vi "2 Global.vi"() -> ()   [LabVIEW 2011]
uses:
  2 Typedefs/UTM Location.ctl
  2 Typedefs/apparent wind.ctl
  2 Typedefs/apparent wind speed.ctl
  2 Typedefs/apparent wind direction.ctl
  2 Typedefs/Velocity.ctl
  2 Typedefs/heading.ctl
  2 Typedefs/generalized actuator status.ctl
  2 Typedefs/indicator LED.ctl
  2 Typedefs/generalized sensor status.ctl
  2 Typedefs/Which Boat.ctl
  2 Typedefs/manual override.ctl
  2 Typedefs/setpoints to boat.ctl
  2 Typedefs/sail setpt.ctl
  2 Typedefs/rudder angle.ctl
panel:
  in  "E-Stop":bool
  in  "Globals":T1(tab)
  in  "Which Boat Am I?":T2 items=["Small RC", "Large RC", "Final Boat", "Simulator"]
  out "Direction Sensor Status":T3
  out "Location Sensor Status":T3
  out "Wind Sensor Status":T3
  out "Sail Actuator Status":T5
  out "Rudder Actuator Status":T5
  in  "Battery Voltage":dbl
  in  "Robot\nHeading":T6 format="%05.1f"
  in  "Robot UTM Location":T7
  in  "Robot Velocity":T8
  out "Overview Image":T9(plugin-control)
  in  "Absolute Wind":T8
  in  "Apparent Wind\nDirection":T10
  in  "Apparent Wind\nSpeed":T11
  in  "Apparent Wind":T12
  in  "Current Destination":T7
  in  "Setpoints to boat":T13
  in  "Manual Override Cluster":T16
  in  "Sail Position":T14
  in  "Rudder Angle":T15
  # "All distances in meters, all speeds in meters per second\nAll angles in degrees, clockwise with 0 being positive North if in global reference frame or 0 being Fore in boat ref frame.\nX-Y make a right handed coordinate system with Z pointing up\nPositive Rudder angle makes the boat turn right\nLocation Coordinates are in UTM format"
  # "As Measured"
  # "From Planning Functions"
  # "Path Planning"
  # "(this is not a cluster because subitems\nare generated in parallel code)"
  # "Mission Definition Stuff Goes HERE"
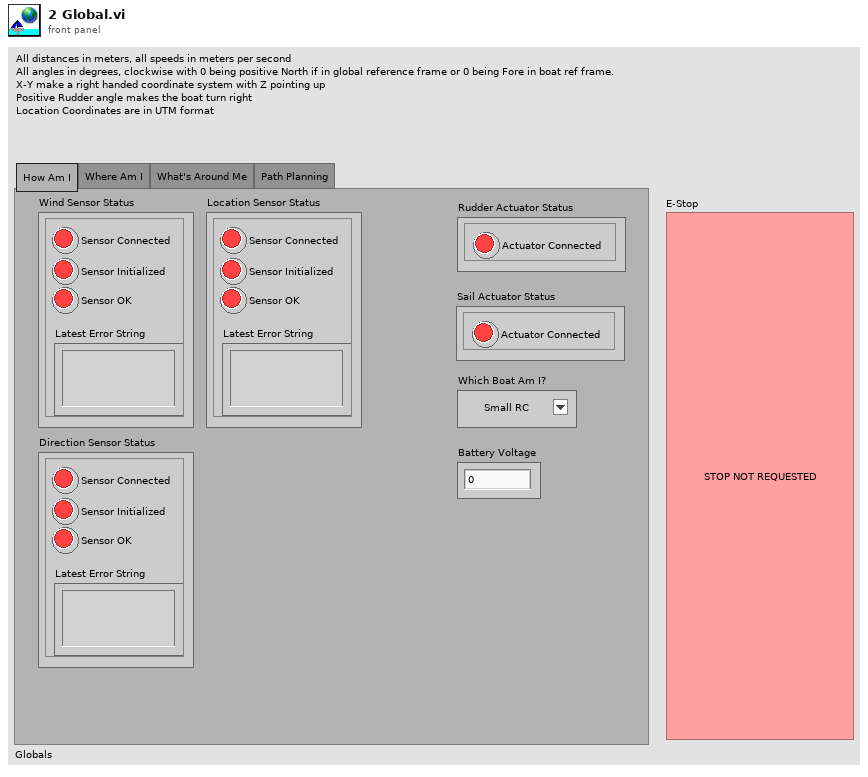
[diagram p1: front panel]
types:
  T1 = enum32{"How Am I", "Where Am I", "What's Around Me", "Path Planning"}
  T2 = typedef "Which Boat.ctl" = u16
  T3 = typedef "generalized sensor status.ctl" = cluster{"Sensor Connected":T4, "Sensor Initialized":T4, "Sensor OK":T4, "Latest Error String":string}
  T4 = typedef "indicator LED.ctl" = bool
  T5 = typedef "generalized actuator status.ctl" = cluster{"Actuator Connected":T4}
  T6 = typedef "heading.ctl" = dbl
  T7 = typedef "UTM Location.ctl" = cluster{"UTM Zone":dbl, "Hemisphere":enum16{"North", "South"}, "East":dbl, "North":dbl}
  T8 = typedef "Velocity.ctl" = cluster{"East":dbl, "North":dbl}
  T9 = typedef "IMAQ Image.ctl" = refnum<image>
  T10 = typedef "apparent wind direction.ctl" = dbl
  T11 = typedef "apparent wind speed.ctl" = dbl
  T12 = typedef "apparent wind.ctl" = cluster{"Toward Fore":dbl, "Toward Starboard":dbl}
  T13 = typedef "setpoints to boat.ctl" = cluster{"Sail Position":T14, "Rudder Angle":T15}
  T14 = typedef "sail setpt.ctl" = dbl
  T15 = typedef "rudder angle.ctl" = dbl
  T16 = typedef "manual override.ctl" = cluster{"Override Active":bool, "Setpoints":T13}
diagram:
